vi "restaurant-tsk4.vi"() -> ()   [LabVIEW 2020]
panel:
  out "Tip Amount":dbl
  in  "Service":bool
  in  "Food":bool
  in  "Stop":bool
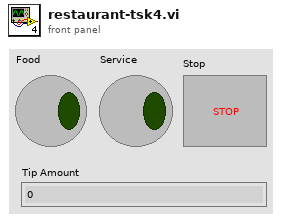
[diagram p1: front panel]
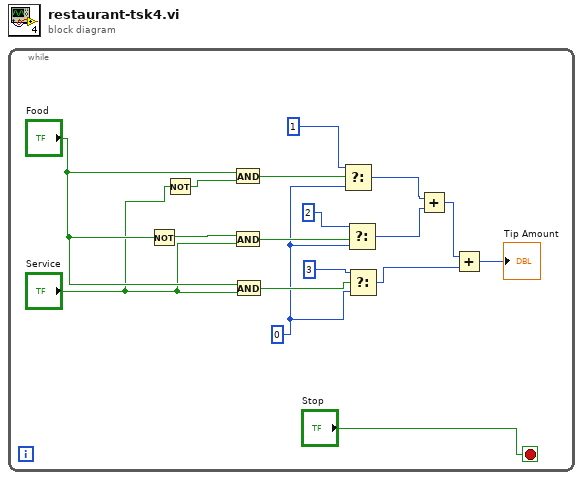
[diagram p0: block diagram]
diagram:
  n1 = while {
    stop <- "Stop" stop-if-true
    w6 = 0
    n2 = Not(x="Food") -> (.not. x?=w16:bool)
    n3 = Not(x="Service") -> (.not. x?=w14:bool)
    n4 = And(x="Food", y=w14) -> (x .and. y?=w12:bool)
    n5 = And(x=w16, y="Service") -> (x .and. y?=w7:bool)
    n6 = And(x="Food", y="Service") -> (x .and. y?=w8:bool)
    n7 = Select(t=1, s=w12, f=w6) -> (s? t:f=w5:i32)
    n8 = Select(t=2, s=w7, f=w6) -> (s? t:f=w4:i32)
    n9 = Select(t=3, s=w8, f=w6) -> (s? t:f=w2:i32)
    n10 = Add(x=w5, y=w4) -> (x+y=w3:i32)
    n11 = Add(x=w3, y=w2) -> (x+y=→"Tip Amount":i32)
  }
